vi "Get Voltage.vi"(8 "error in":errorcluster, 11 "DMA in":refnum<class "DMA.lvclass">) -> (0 "error out":errorcluster, 2 "V":dbl, 3 "DMA out":refnum<class "DMA.lvclass">)   [LabVIEW 2015, in "DMA.lvclass"]
uses:
  DMA.lvclass
  DMA.lvclass/DMA.ctl
  Accessors/Read Gas Ref.vi
  Accessors/Read Qex.vi
  Accessors/Read Qsh.vi
  Accessors/Read ro.vi
  Accessors/Read ri.vi
  Accessors/Read Leff.vi
  Accessors/Read Particle.vi
  Particle Class/Calculate Electric Mobility.vi
  Atmospheric/Gas Properties/Gas Properties.lvclass
  Particle Class/Particle Properties.lvclass
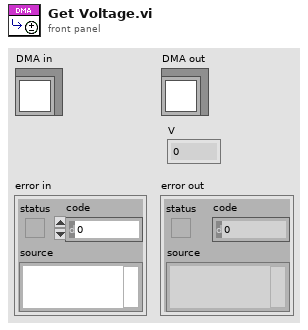
[diagram p1: front panel]
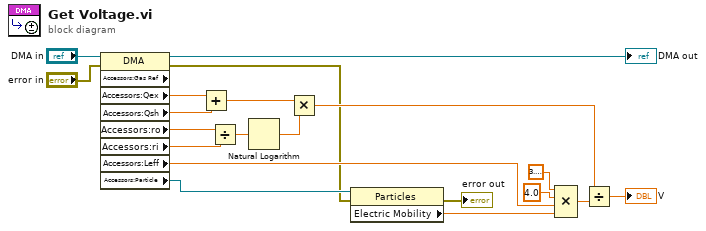
[diagram p0: block diagram]
diagram:
  n1 = property class="DMA" props=["Accessors:Gas Ref", "Accessors:Qex", "Accessors:Qsh", "Accessors:ro", "Accessors:ri", "Accessors:Leff", "Accessors:Particle"](reference="DMA in", error in="error in") -> (reference out=→"DMA out":refnum<class "DMA.lvclass">, error out=w3:errorcluster, "Accessors:Qex"=w19:dbl, "Accessors:Qsh"=w18:dbl, "Accessors:ro"=w17:dbl, "Accessors:ri"=w16:dbl, "Accessors:Leff"=w12:dbl, "Accessors:Particle"=w7:refnum<class "Particle Properties.lvclass">)  [unwired: 1 out]
  n2 = Add(x=w19, y=w18) -> (x+y=w10:dbl)
  n3 = Divide(x=w17, y=w16) -> (x/y=w15:dbl)
  n4 = Natural Logarithm(1:w15) -> (0:w9:dbl)
  n5 = Multiply(x=w10, y=w9) -> (x*y=w8:dbl)
  n6 = property class="Particles"(reference=w7, error in=w3) -> (error out=→"error out":errorcluster, "Electric Mobility"=w6:dbl)  [unwired: 1 out]
  n7 = Compound Arithmetic op=MULTIPLY(3.141592653589793, 4.0 ("x"), w12, w6) -> (w11:dbl)
  n8 = Divide(x=w8, y=w11) -> (x/y=→"V":dbl)
